vi "New Image.vi"   [LabVIEW 2011, in "labvvis.lvlib"]
doc: "Creates a new image."
uses:
  <userlib>/labvvis/labvvis.lvlib
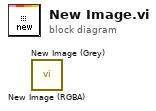
[diagram p0: block diagram]
diagram:
  n1 = call <userlib>:"New Image (RGBA).vi"() -> ()  [unwired: 4 in, 2 out]
  n2 = call <userlib>:"New Image (Grey).vi"() -> ()  [unwired: 4 in, 2 out]
